vi "Odd bit extractor.vi"() -> ()   [LabVIEW 2026]
panel:
  out "Odd bits":i8
  in  "Loop Index":i8
  in  "input PN Sequence":i8[](array[numeric])
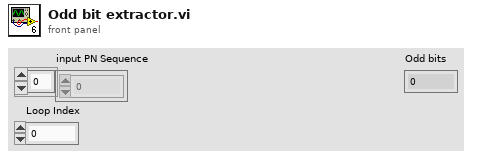
[diagram p1: front panel]
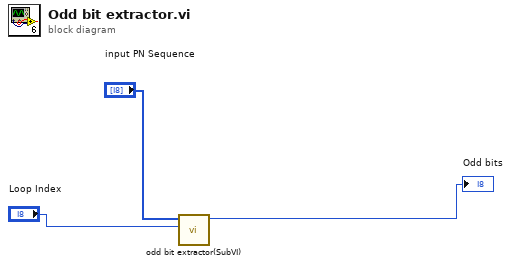
[diagram p0: block diagram]
diagram:
  n1 = call "odd bit extractor(SubVI).vi"("Loop Index"="Loop Index", "input PN Sequence"="input PN Sequence") -> ("Odd bits"=→"Odd bits":i8)  [unwired: 9 in]
